vi "GetisciFilemeasures_settings_OUTPUT.vi"(4 "Azione":string, 9 "banco":i32, 10 "Array ClusterCaratteristicheMisura IN":T1[](array[typedef]), 11 "Numero Misure":dbl) -> (2 "Array ClusterCaratteristicheMisura OUT":T1[](array[typedef]))   [LabVIEW 2019]
uses:
  TypeDef/ClusterCaratteristicheMisura_OUTPUT.ctl
  <vilib>/Utility/file.llb/Read Delimited Spreadsheet (string).vi
panel:
  in  "Cluster Caratteriestiche Misura":T1
  out "Lettura file txt":string[][](array[string])
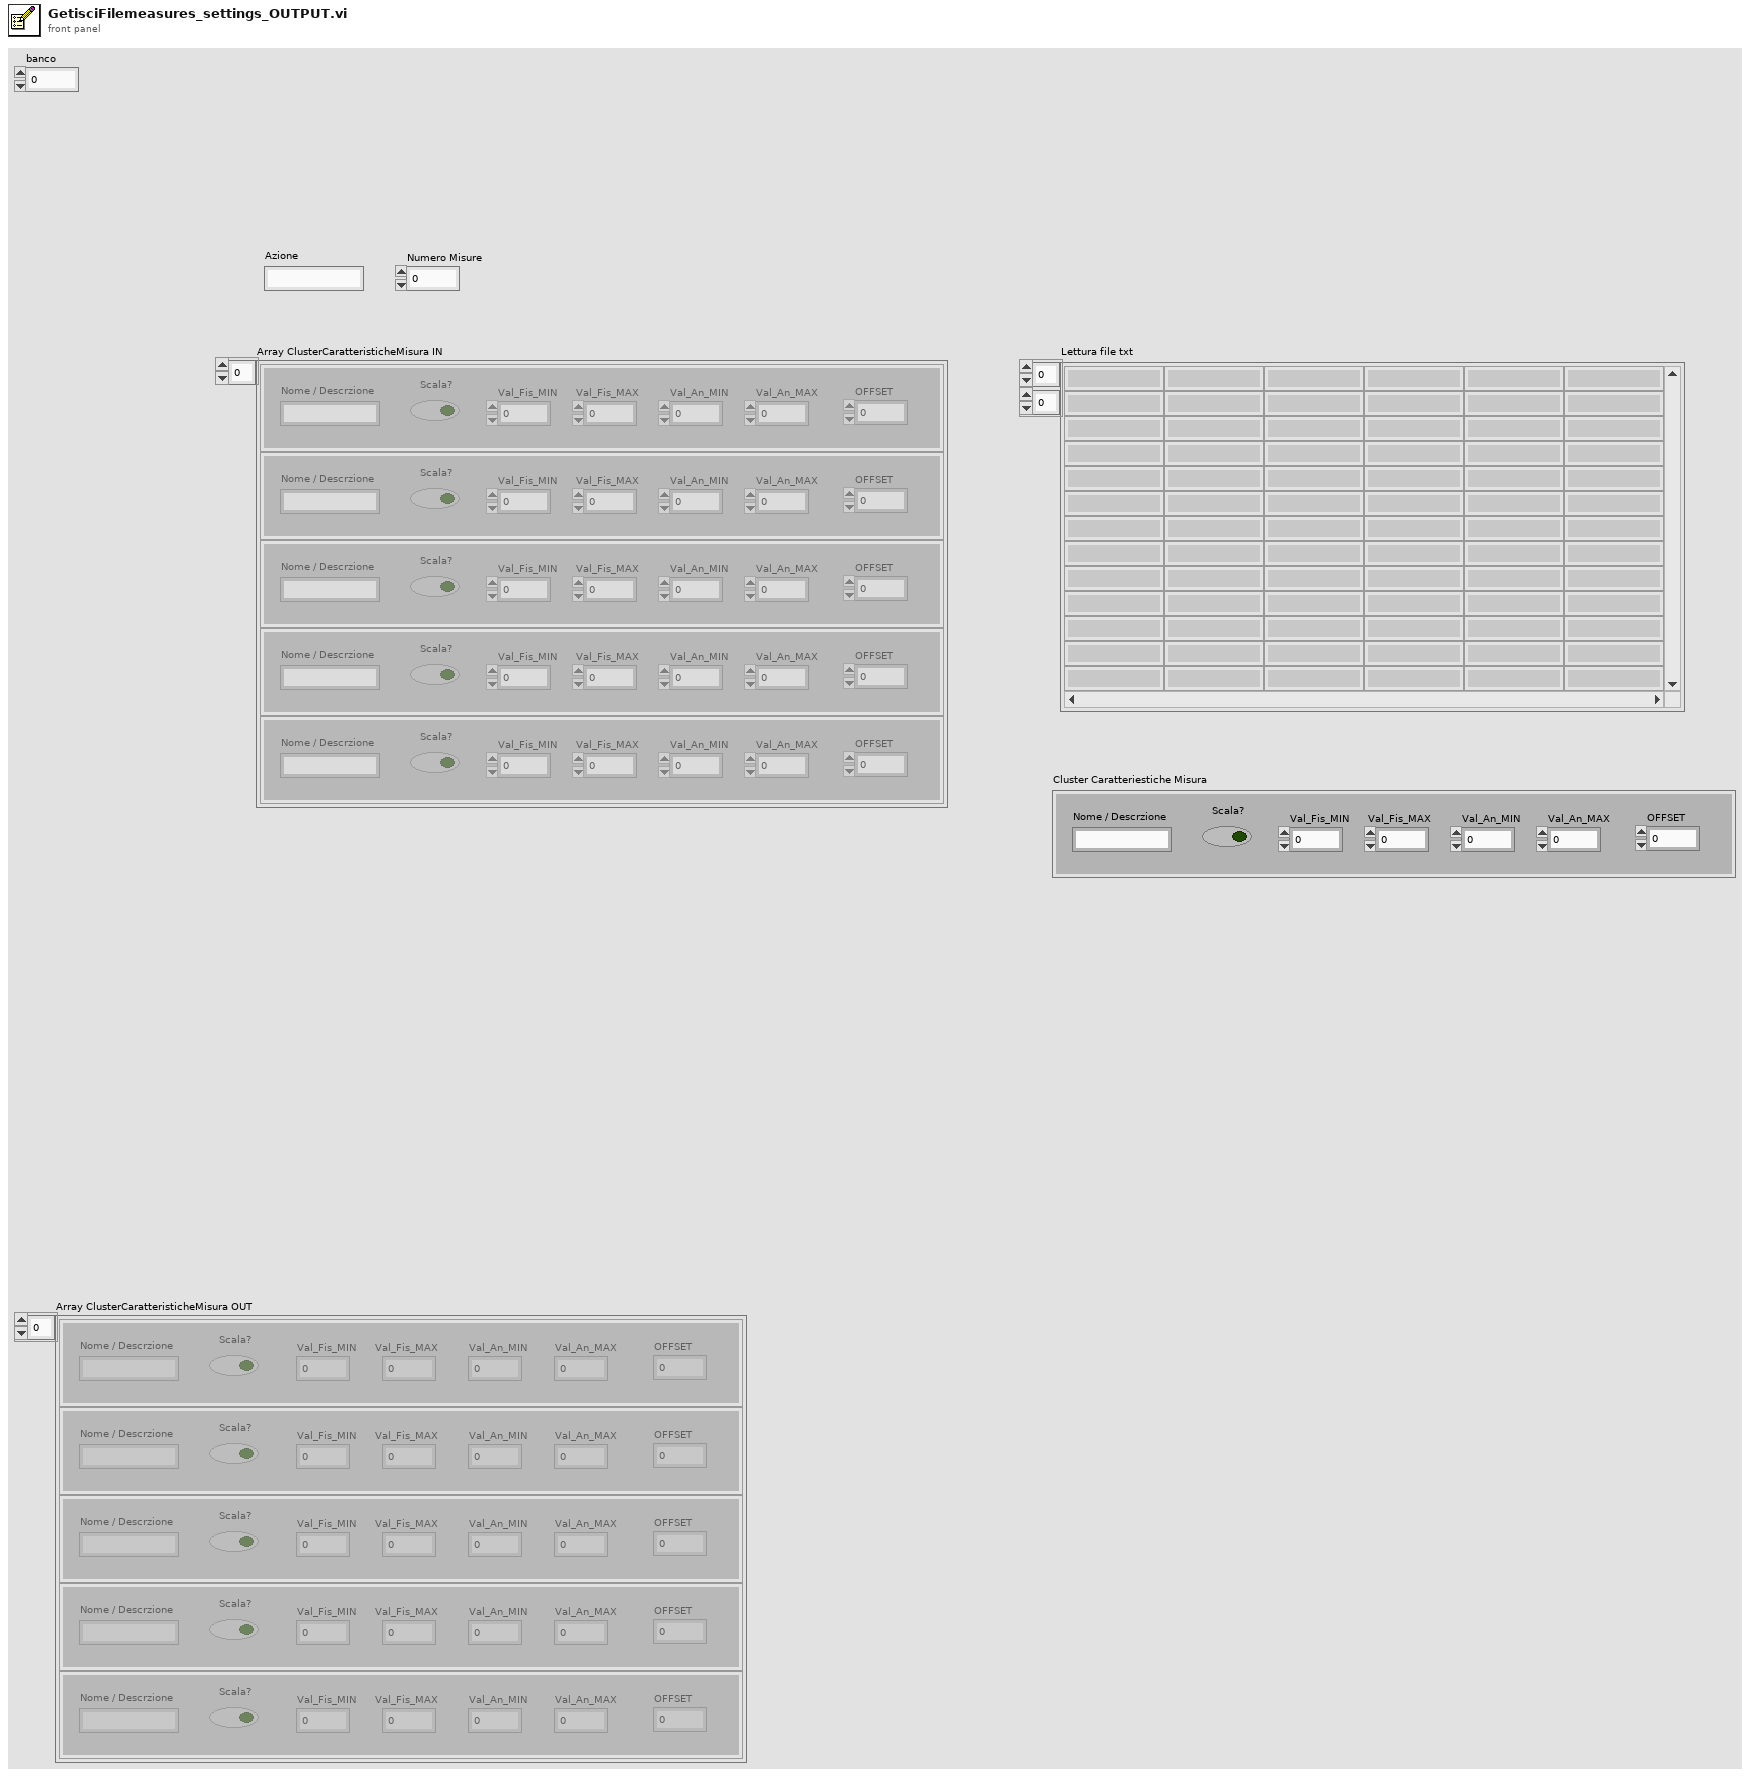
[diagram p1: front panel]
types:
  T1 = typedef "ClusterCaratteristicheMisura_OUTPUT.ctl" = cluster{"Nome / Descrzione":string, "Scala?":bool, "Val_Fis_MIN":dbl, "Val_Fis_MAX":dbl, "Val_An_MIN":dbl, "Val_An_MAX":dbl, "OFFSET":dbl}
  T2 = enum16{"open", "replace", "create", "open or create", "replace or create", "replace or create with confirmation"}
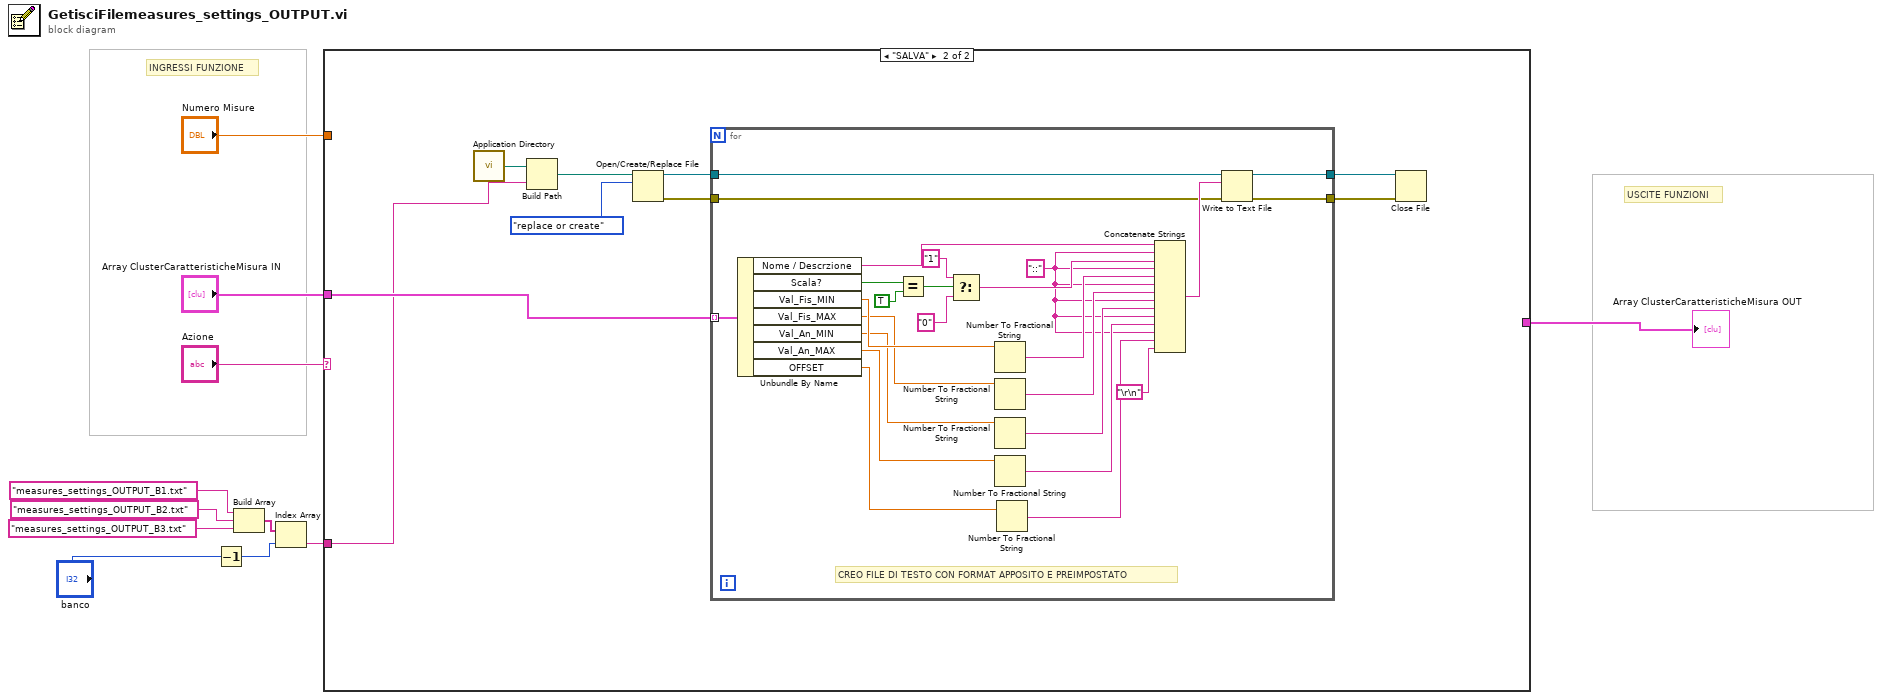
[diagram p0: block diagram]
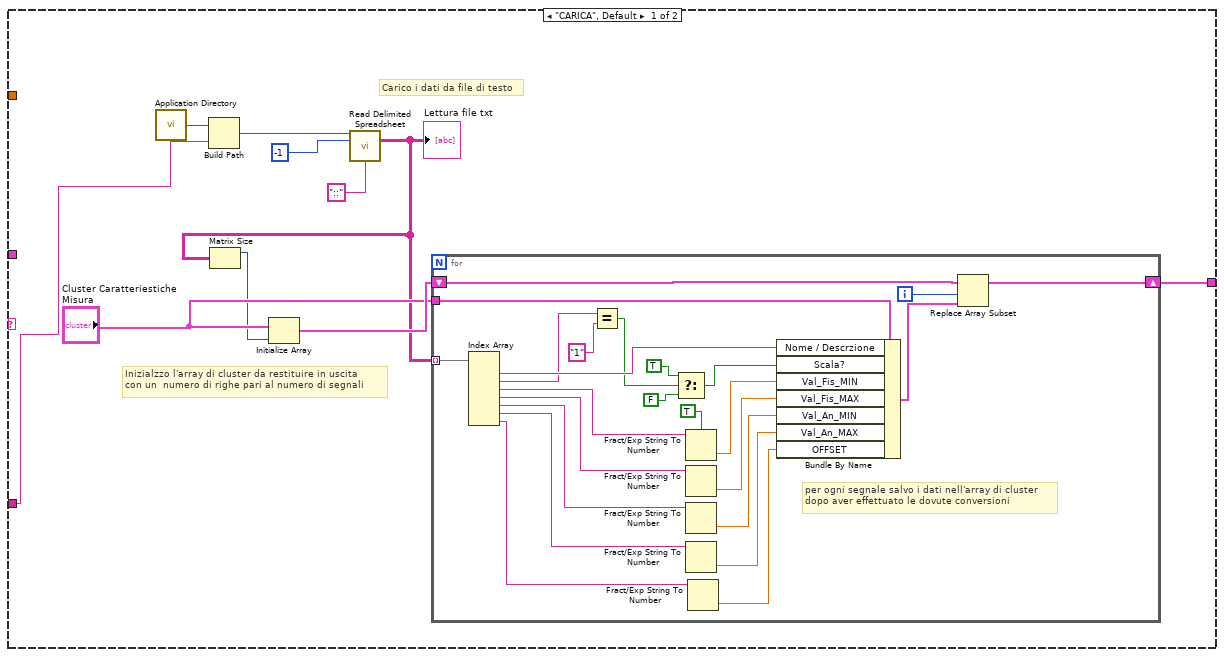
[diagram p2: hidden frame]
diagram:
  # "USCITE FUNZIONI"
  # "INGRESSI FUNZIONE"
  n1 = Decrement(x="banco") -> (x-1=w8:i32)
  n2 = Build Array("measures_settings_OUTPUT_B1.txt" ("name or relative path"), "measures_settings_OUTPUT_B2.txt" ("name or relative path"), "measures_settings_OUTPUT_B3.txt" ("name or relative path")) -> (w7:string[])
  n3 = Index Array(array=w7, index=w8) -> (element=w2:string)
  n4 = case shown="\"SALVA\"" "Azione" {
    tunnel: "Array ClusterCaratteristicheMisura IN" -> [_ w47]
    tunnel: "Numero Misure" -> [_ _]
    tunnel: [w16 _] -> w1
    tunnel: w2 -> [w12 w46]
    frame "CARICA", Default {
      # "Inizialzzo l'array di cluster da restituire in uscita\ncon un  numero di righe pari al numero di segnali"
      # "Carico i dati da file di testo"
      n5 = call <vilib>:"Application Directory.vi"() -> ("Application Directory"=w21:path)
      n6 = Build Path(base path=w21, name or relative path=w12) -> (appended path=w20:path)
      n7 = call-poly <vilib>:"Read Delimited Spreadsheet.vi"("file path (dialog if empty)"=w20, "number of rows (all:-1)"=-1, "delimiter (\\t)"="::" ("delimiter (\\t)")) -> ("all rows"=w14:string[][])  [unwired: 7 in, 5 out]
      "Lettura file txt" <- w14
      n8 = Matrix Size(0:w14) -> (1:w13:i32)  [unwired: 1 out]
      n9 = Initialize Array("Cluster Caratteriestiche Misura", w13) -> (w17:T1[])
      n10 = for {
        tunnel: w14 -> [w45] mode=indexing
        tunnel: "Cluster Caratteriestiche Misura" -> [w26]
        shift-right: [w22] -> w16
        shift-left: w17 -> [w25]
        i -> [w23]
        # "per ogni segnale salvo i dati nell'array di cluster \ndopo aver effettuato le dovute conversioni"
        n11 = Index Array(array=w45) -> (element #1=w44:string, element #2=w43:string, element #3=w36:string, element #4=w34:string, element #5=w33:string, element #6=w32:string, element #7=w28:string)  [unwired: 7 in]
        n12 = Equal?(x=w43, y="1") -> (x = y?=w41:bool)
        n13 = Select(t=TRUE, s=w41, f=FALSE) -> (s? t:f=w38:bool)
        n14 = Fract/Exp String To Number(use system decimal point (T)=TRUE, string=w36) -> (number=w35:dbl)  [unwired: 2 in, 1 out]
        n15 = Fract/Exp String To Number(string=w34) -> (number=w31:dbl)  [unwired: 3 in, 1 out]
        n16 = Fract/Exp String To Number(string=w33) -> (number=w30:dbl)  [unwired: 3 in, 1 out]
        n17 = Fract/Exp String To Number(string=w32) -> (number=w29:dbl)  [unwired: 3 in, 1 out]
        n18 = Fract/Exp String To Number(string=w28) -> (number=w27:dbl)  [unwired: 3 in, 1 out]
        n19 = Bundle By Name(cluster=w26, "Nome / Descrzione"=w44, "Scala?"=w38, "Val_Fis_MIN"=w35, "Val_Fis_MAX"=w31, "Val_An_MIN"=w30, "Val_An_MAX"=w29, "OFFSET"=w27) -> (w24:T1)
        n20 = Replace Array Subset(array=w25, new element=w24, index=w23) -> (w22:T1[])
      }
    }
    frame "SALVA" {
      n21 = call <vilib>:"Application Directory.vi"() -> ("Application Directory"=w54:path)
      n22 = Build Path(base path=w54, name or relative path=w46) -> (appended path=w52:path)
      n23 = Open/Create/Replace File(file path (use dialog)=w52, operation (0:open)=T2."replace or create") -> (refnum out=w53:refnum<file>, error out=w49:errorcluster)  [unwired: 4 in, 1 out]
      n24 = for {
        tunnel: w53 -> [w78]
        tunnel: w47 -> [w79] mode=indexing
        tunnel: [w66] -> w50
        tunnel: w49 -> [w65]
        tunnel: [w64] -> w48
        w58 = "::" ("string")
        # "CREO FILE DI TESTO CON FORMAT APPOSITO E PREIMPOSTATO"
        n25 = Unbundle By Name(w79) -> ("Nome / Descrzione"=w72:string, "Scala?"=w77:bool, "Val_Fis_MIN"=w71:dbl, "Val_Fis_MAX"=w70:dbl, "Val_An_MIN"=w69:dbl, "Val_An_MAX"=w68:dbl, "OFFSET"=w56:dbl)
        n26 = Equal?(x=w77, y=TRUE) -> (x = y?=w75:bool)
        n27 = Select(t="1", s=w75, f="0") -> (s? t:f=w63:string)
        n28 = Number To Fractional String(number=w71) -> (F-format string=w62:string)  [unwired: 3 in]
        n29 = Number To Fractional String(number=w70) -> (F-format string=w61:string)  [unwired: 3 in]
        n30 = Number To Fractional String(number=w69) -> (F-format string=w60:string)  [unwired: 3 in]
        n31 = Number To Fractional String(number=w68) -> (F-format string=w59:string)  [unwired: 3 in]
        n32 = Number To Fractional String(number=w56) -> (F-format string=w55:string)  [unwired: 3 in]
        n33 = Concatenate Strings(w72, w58, w63, w58, w62, w58, w61, w58, w60, w58, w59, w58, w55, "\r\n") -> (w67:string)
        n34 = Write to Text File(file (use dialog)=w78, text=w67, error in=w65) -> (refnum out=w66:refnum<file>, error out=w64:errorcluster)  [unwired: 1 in, 1 out]
      }
      n35 = Close File(refnum=w50, error in=w48) -> ()  [unwired: 2 out]
    }
  }
  "Array ClusterCaratteristicheMisura OUT" <- w1
